vi "测量平均周期.vi"(9 "运行总次数（为0则一直进行）":u32, 10 "已运行次数（i+1）":i32, 11 "初始时间":u32) -> (2 "布尔":bool, 3 "平均周期":dbl)   [LabVIEW 2018]
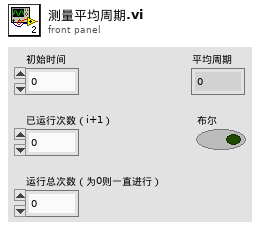
[diagram p1: front panel]
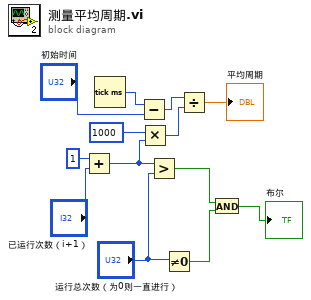
[diagram p0: block diagram]
diagram:
  n1 = Add(x=u32 1 ("y"), y="已运行次数（i+1）") -> (x+y=w13:u32)
  n2 = Tick Count (ms)() -> (millisecond timer value=w5:u32)
  n3 = Subtract(x=w5, y="初始时间") -> (x-y=w7:u32)
  n4 = Multiply(x=u32 1000 ("y"), y=w13) -> (x*y=w10:u32)
  n5 = Greater?(x=w13, y="运行总次数（为0则一直进行）") -> (0:w3:bool)
  n6 = Not Equal To 0?(x="运行总次数（为0则一直进行）") -> (x != 0?=w2:bool)
  n7 = Divide(x=w7, y=w10) -> (x/y=→"平均周期":dbl)
  n8 = And(x=w3, y=w2) -> (x .and. y?=→"布尔":bool)
